vi "Set Output Res.vi"(0 "COM Port":string="COM3", 5 "Resistance":dbl=1900.0, 7 "Delay Time (s)":string, 9 "Output Type":i32(ring)=8 items=["DC Volts", "AC Volts", "DC Current", "AC Current", "DC Power", "AC Power", "Dual DC Volts", "Dual AC Volts", "Resistance"], 11 "error in":errorcluster, 12 "Output Enabled":bool) -> (15 "error out":errorcluster)   [LabVIEW 2013]
uses:
  <instrlib>/Fluke 5080/Fluke 5080.lvlib
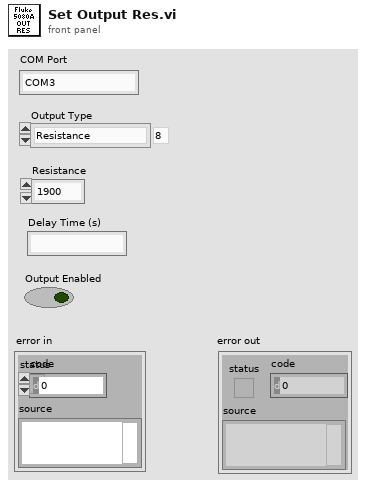
[diagram p1: front panel]
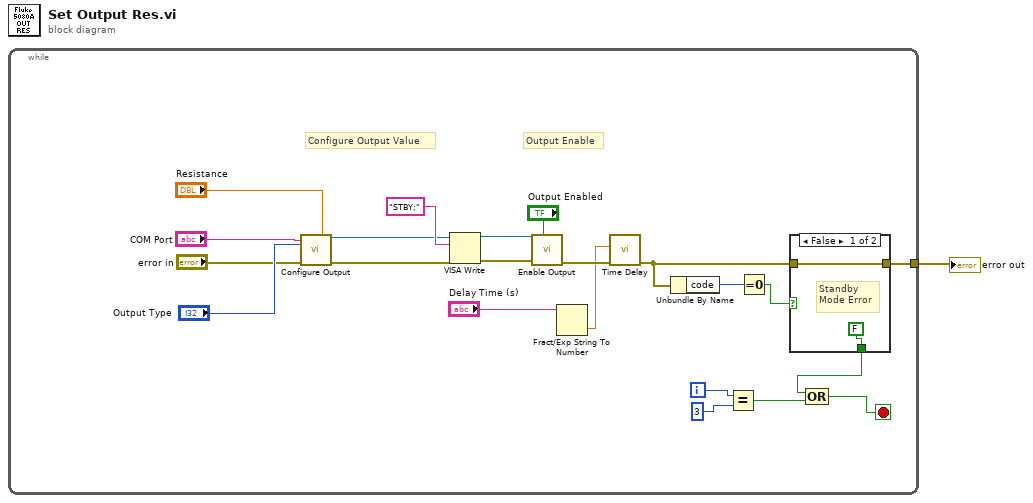
[diagram p0: block diagram]
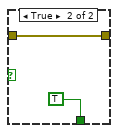
[diagram p2: hidden frame]
diagram:
  n1 = while {
    tunnel: [w9] -> w1
    i -> [w14]
    stop <- w11 stop-if-true
    # "Output Enable"
    # "Configure Output Value"
    n2 = call <instrlib>:"Configure Output.vi"("VISA resource name"="COM Port", "Resistance (1900.0 Ohm)"="Resistance", "Output Type (0: DC Volts)"="Output Type", "error in (no error)"="error in") -> ("VISA resource name out"=w5:refnum<visa-resource-name>, "error out"=w4:errorcluster)  [unwired: 6 in, 4 out]
    n3 = VISA Write(VISA resource name=w5, write buffer="STBY;", error in (no error)=w4) -> (VISA resource name out=w20:refnum<visa-resource-name>, error out=w19:errorcluster)  [unwired: 1 out]
    n4 = call <instrlib>:"Enable Output.vi"("Output Enabled (T: Enable)"="Output Enabled", "error in (no error)"=w19, "VISA resource name"=w20) -> ("error out"=w21:errorcluster)  [unwired: 8 out]
    n5 = Fract/Exp String To Number(string="Delay Time (s)") -> (number=w2:dbl)  [unwired: 3 in, 1 out]
    n6 = call "Time Delay"("error in (no error)"=w21, "Delay Time (s)"=w2) -> ("error out"=w10:errorcluster)  [unwired: 9 in]
    n7 = Unbundle By Name(w10) -> ("code"=w17:i32)
    n8 = Equal?(x=w14, y=3) -> (x = y?=w12:bool)
    n9 = Equal To 0?(x=w17) -> (x = 0?=w16:bool)
    n10 = case shown="False" w16 {
      tunnel: [FALSE TRUE] -> w13
      tunnel: w10 -> [w24 w26]
      tunnel: [w24 w26] -> w9
      frame False {
        # "Standby\nMode Error"
      }
      frame True {
      }
    }
    n11 = Compound Arithmetic op=OR(w13, w12) -> (w11:bool)
  }
  "error out" <- w1
